vi "Read TCPSettings.vi"(8 "error in (no error)":errorcluster, 11 "TCPCommunicator in":refnum<class "TCPCommunicator.lvclass">) -> (0 "error out":errorcluster, 2 "TCPSettings.lvclass":refnum<class "TCPSettings.lvclass">, 3 "TCPCommunicator out":refnum<class "TCPCommunicator.lvclass">)   [LabVIEW 2016, in "TCPCommunicator.lvclass"]
uses:
  TCPCommunicator.lvclass
  TCPSettings/TCPSettings.lvclass
  TCPCommunicator.lvclass/TCPCommunicator.ctl
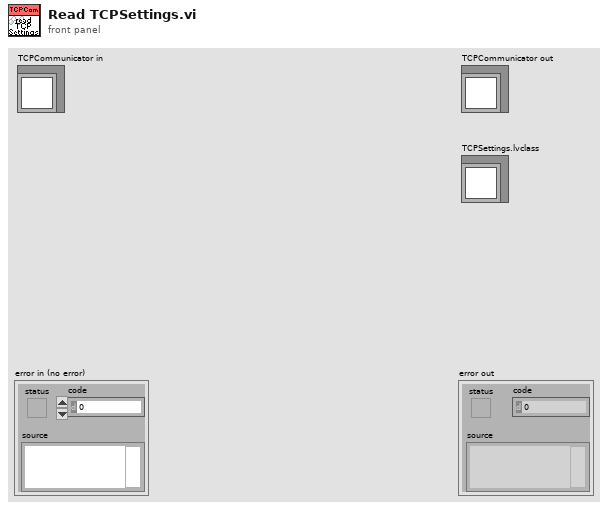
[diagram p1: front panel]
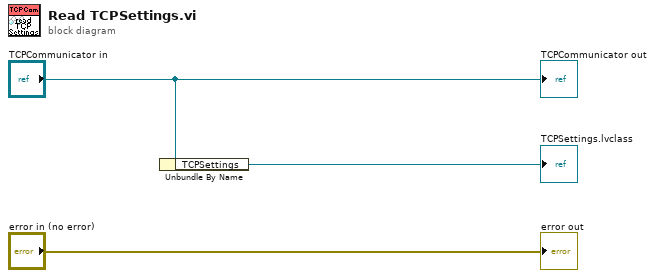
[diagram p0: block diagram]
diagram:
  n1 = Unbundle By Name("TCPCommunicator in") -> ("TCPSettings"=→"TCPSettings.lvclass":refnum<class "TCPSettings.lvclass">)
  "error out" <- "error in (no error)"
  "TCPCommunicator out" <- "TCPCommunicator in"
